vi "StopCapture.vi"(8 "error in (no error)":errorcluster, 11 "Inovance_Camera in":refnum<class "Inovance_Camera.lvclass">) -> (0 "error out":errorcluster, 3 "Inovance_Camera out":refnum<class "Inovance_Camera.lvclass">)   [LabVIEW 2023, in "CameraLibrary.lvlib" / "Inovance_Camera.lvlib" / "Inovance_Camera.lvclass"]
uses:
  Inovance_Camera.lvclass
  C:/Program Files/National Instruments/LabVIEW 2023/vi.lib/ActorFramework/Actor/Actor.lvclass
  <vilib>/userDefined/High Color/IMAQdx.ctl
  <vilib>/ActorFramework/Actor/Actor.lvclass/Actor.ctl
  Inovance_Camera.lvclass/Inovance_Camera.ctl
  <vilib>/ActorFramework/Message Enqueuer/Message Enqueuer.lvclass/Message Enqueuer.ctl
  <vilib>/ActorFramework/Message Enqueuer/Enqueue.vi
  Interfaces/AbstractInstrumentClasses/Cameras_LV/CameraComm Messages/Capture Stopped Msg/Capture Stopped Msg.lvclass
  C:/Program Files/National Instruments/LabVIEW 2023/vi.lib/ActorFramework/Message/Message.lvclass
  <vilib>/ActorFramework/Message Priority Queue/Priority Enqueue.vi
  <vilib>/vision/driver/NI_Vision_Acquisition_Software.lvlib
  <vilib>/ActorFramework/Actor/Actor.lvclass
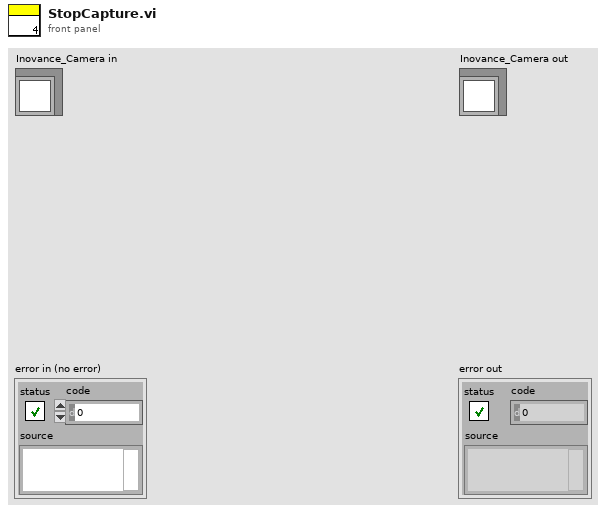
[diagram p1: front panel]
types:
  T1 = typedef "IMAQdx.ctl" = refnum<k21>
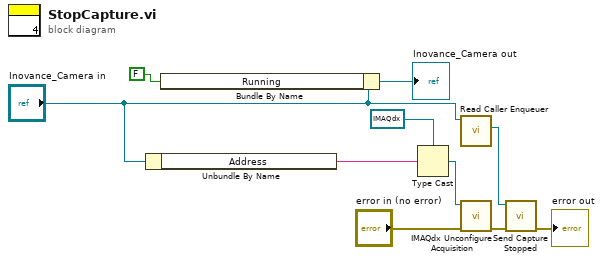
[diagram p0: block diagram]
diagram:
  n1 = Unbundle By Name("Inovance_Camera in") -> ("Address"=w5:string)
  n2 = Bundle By Name(cluster="Inovance_Camera in", "Running"=FALSE ("InstrumentData.CurrentState.Connected")) -> (→"Inovance_Camera out":refnum<class "Inovance_Camera.lvclass">)
  n3 = Type Cast(type=T1 refnum ("Inovance Address"), x=w5) -> (*(type *) &x=w4:T1)
  n4 = call <vilib>:"Read Caller Enqueuer.vi"("Actor"="Inovance_Camera in") -> ("Caller Enqueuer"=w9:refnum<class "Message Enqueuer.lvclass">)  [unwired: 10 in]
  n5 = call <vilib>:"IMAQdx Unconfigure Acquisition.vi"("error in"="error in (no error)", "Session In"=w4) -> ("error out"=w8:errorcluster)  [unwired: 8 in, 1 out]
  n6 = call "Send Capture Stopped.vi"("error in (no error)"=w8, "Message Enqueuer"=w9) -> ("error out"=→"error out":errorcluster)  [unwired: 8 in, 1 out]
